vi "Get FPGA uService ID.vi"(6 "error in (no error)":errorcluster, 8 "Kasli Name":string, 9 "Kasli in":refnum<class "Kasli.lvclass">) -> (0 "error out":errorcluster, 1 "uService ID":string, 2 "uService Class Name":string)   [LabVIEW 2020, in "Kasli Wrapper 2.0.lvlib" / "Kasli.lvclass"]
uses:
  Kasli.lvclass
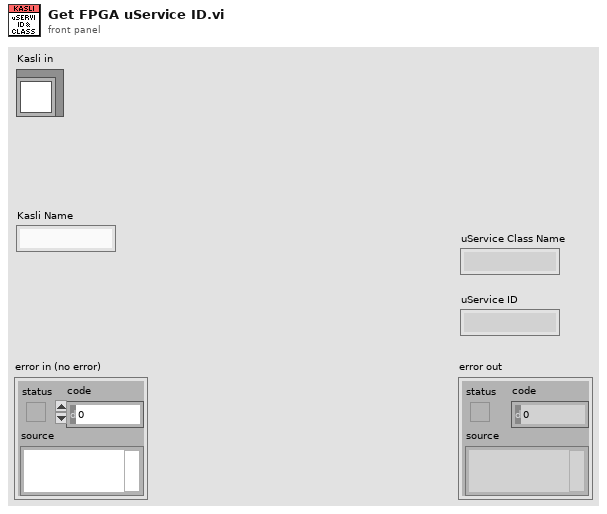
[diagram p1: front panel]
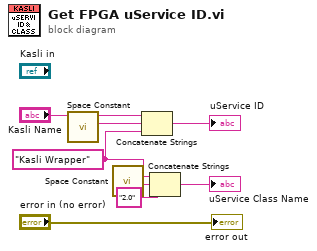
[diagram p0: block diagram]
diagram:
  w4 = "Kasli Wrapper" ("uService Class name")
  n1 = call <vilib>:"Space Constant.vi"() -> ("String"=w6:string)
  n2 = call <vilib>:"Space Constant.vi"() -> ("String"=w3:string)
  n3 = Concatenate Strings("Kasli Name", w6, w4) -> (→"uService ID":string)
  n4 = Concatenate Strings(w4, w3, "2.0" ("string")) -> (→"uService Class Name":string)
  "error out" <- "error in (no error)"
